vi "serial_read.vi"(4 "错误输入（无错误）":errorcluster, 5 "VISA资源名称":refnum<visa-resource-name>) -> (0 "错误输出":errorcluster, 1 "读取缓冲区":string, 2 "VISA资源名称输出":refnum<visa-resource-name>)   [LabVIEW 2020]
panel:
  out "错误输出 2":errorcluster caption="错误输出"
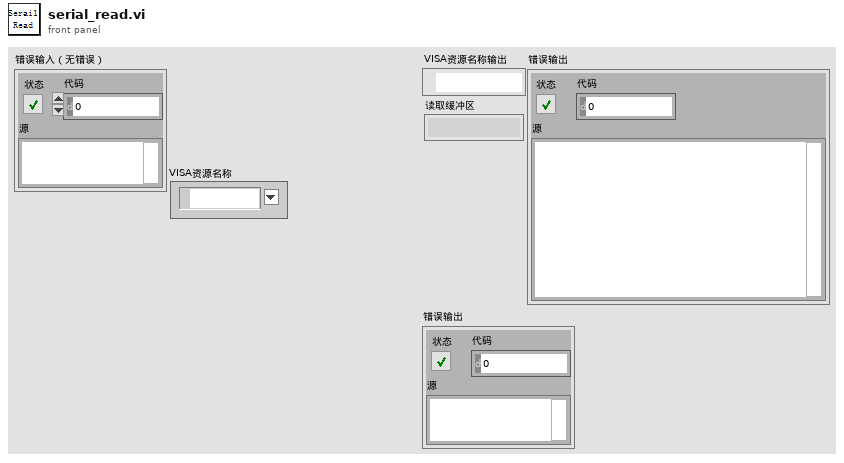
[diagram p1: front panel]
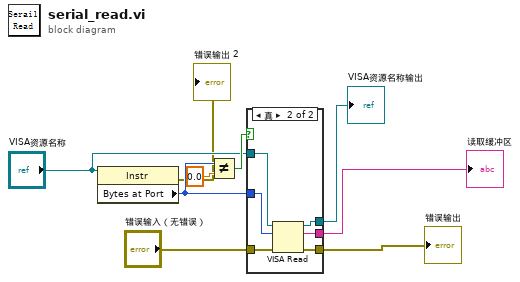
[diagram p0: block diagram]
diagram:
  n1 = property class="Instr"(reference="VISA资源名称") -> (error out=→"错误输出 2":errorcluster, "Bytes at Port"=w2:u32)  [unwired: 1 in, 1 out]
  n2 = Not Equal?(x=w2, y=0.0) -> (x != y?=w8:bool)
  n3 = case shown="真" w8 {
    tunnel: "错误输入（无错误）" -> [_ w15]
    tunnel: "VISA资源名称" -> [_ w14]
    tunnel: [_ w13] -> w5
    tunnel: [_ w12] -> w4
    tunnel: [_ w11] -> w3
    tunnel: w2 -> [_ w10]
    frame False {
    }
    frame True {
      n4 = VISA Read(VISA resource name=w14, byte count=w10, error in (no error)=w15) -> (VISA resource name out=w11:refnum<visa-resource-name>, read buffer=w12:string, error out=w13:errorcluster)  [unwired: 1 out]
    }
  }
  "VISA资源名称输出" <- w3
  "读取缓冲区" <- w4
  "错误输出" <- w5
